vi "IR and Dielectric Strength Test.vi"(0 "VISA resource name in":refnum<visa-resource-name>="COM12", 11 "error in (no error)":errorcluster) -> (2 "Stop Status":bool, 3 "Stop Status":string, 4 "BW 1 Results":T2, 6 "BW 2 Results":T2, 8 "Raw Data ACW BW1":T4, 10 "Raw Data ACW BW2":T3, 13 "BW1 Result Indicators":T1, 14 "BW2 Result Indicators":T1, 15 "error out":errorcluster)   [LabVIEW 2018]
uses:
  Custom Controls/Vitrek State Variable.ctl
  <vilib>/Instr/_visa.llb/VISA Configure Serial Port (Instr).vi
  Door Status Global Variable.vi
panel:
  in  "Insulation Resistance (Mohms)":dbl=100.0 format="%#_13g"
  in  "Dielectric Strength (uA)":dbl=50.0 format="%#_13g"
  out "Test Status":string
  out "Dielectric Strength Voltage - BW2":dbl[](graph)
  out "Dielectric Strength Current - BW2":dbl[](graph)
  out "Dielectric Strength Current - BW1":dbl[](graph)
  out "Dielectric Strength Voltage - BW1":dbl[](graph) caption="Dielectric Strength Voltage Test 1"
  out "Test Results":string
  out "Current Step":string
  in  "Vitrek States":T5=enum."Config ACW Bridgewire 1"
  # "Bridgewire 1"
  # "Bridgewire 2"
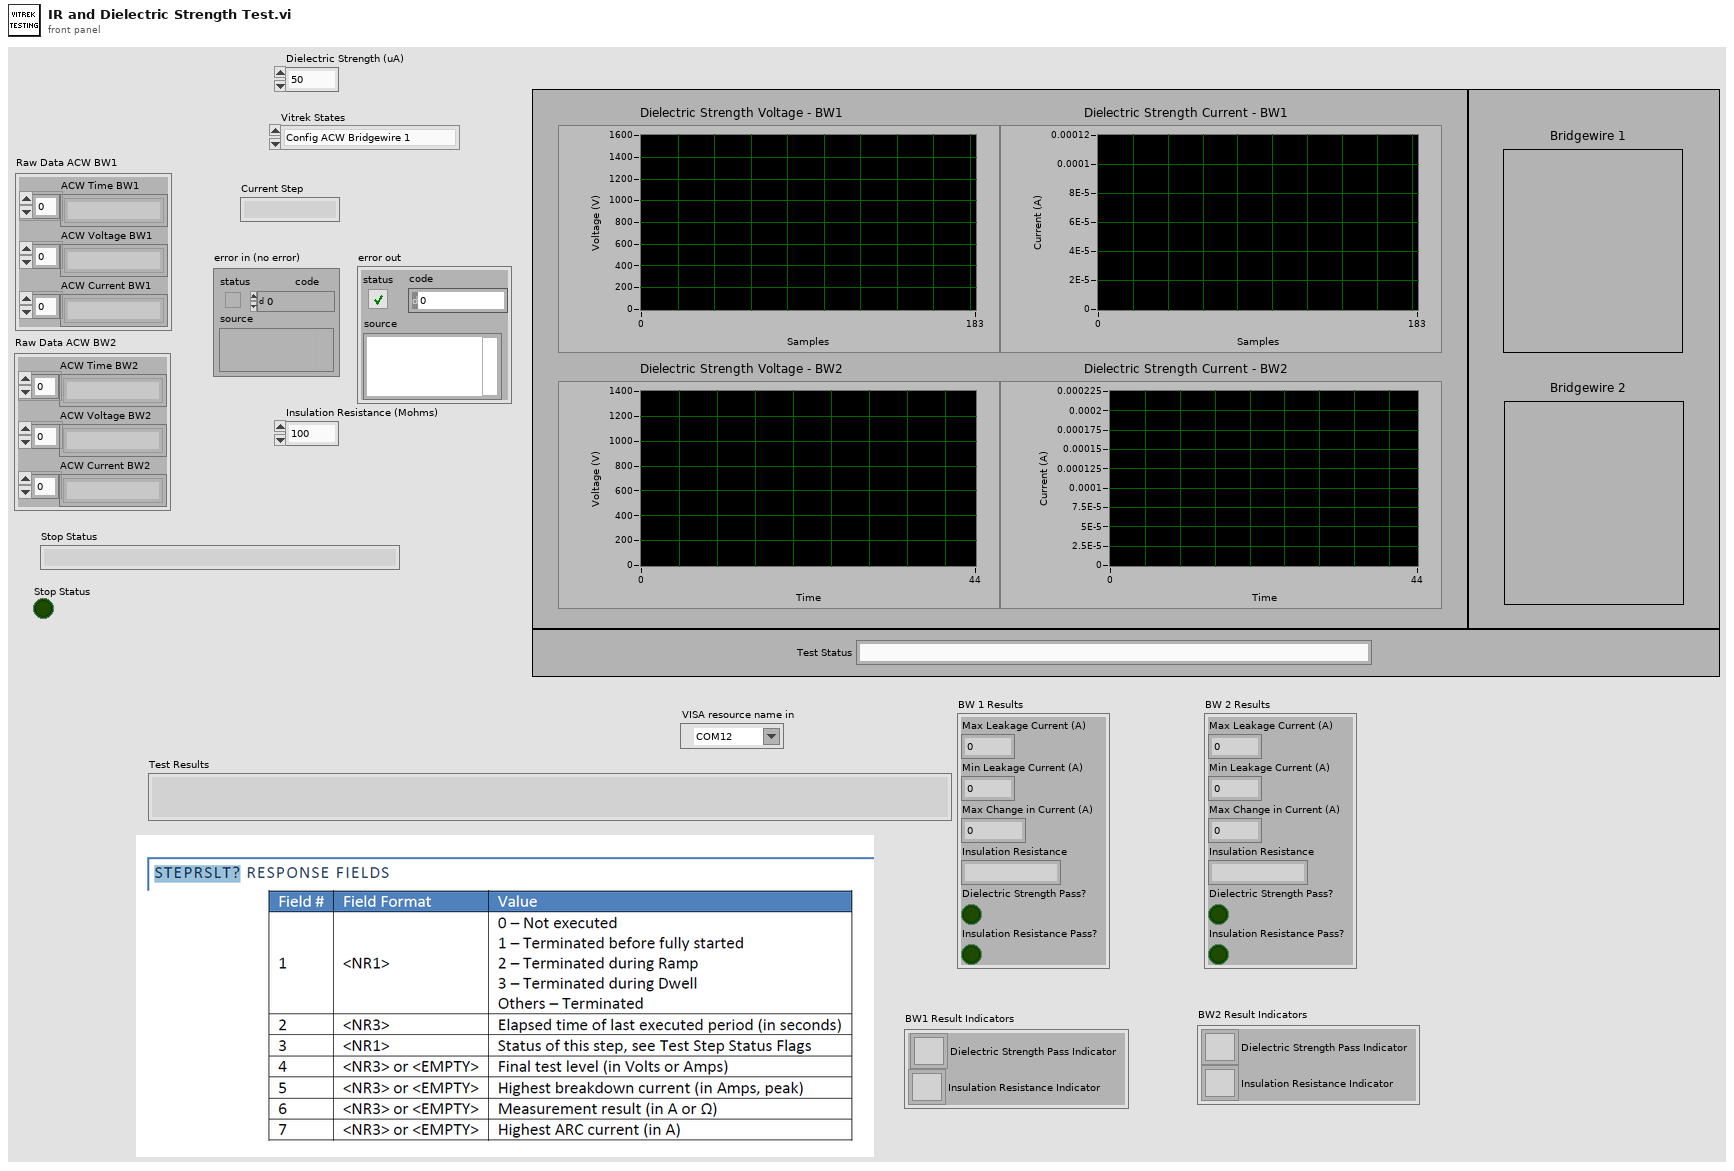
[diagram p1: front panel]
types:
  T1 = cluster{"Dielectric Strength Pass Indicator":u16, "Insulation Resistance Indicator":u16}
  T2 = cluster{"Max Leakage Current (A)":dbl, "Min Leakage Current (A)":dbl, "Max Change in Current (A)":dbl, "Dielectric Strength Pass?":bool, "Insulation Resistance Pass?":bool, "Insulation Resistance":string}
  T3 = cluster{"ACW Time BW2":string[], "ACW Voltage BW2":string[], "ACW Current BW2":string[]}
  T4 = cluster{"ACW Time BW1":string[], "ACW Voltage BW1":string[], "ACW Current BW1":string[]}
  T5 = typedef "Vitrek State Variable.ctl" = enum16{"Clear Tests", "Config ACW Bridgewire 1", "Config ACW Bridgewire 2", "Config IR Bridgewire 1", "Config IR Bridgewire 2", "Run Test", "Stop"}
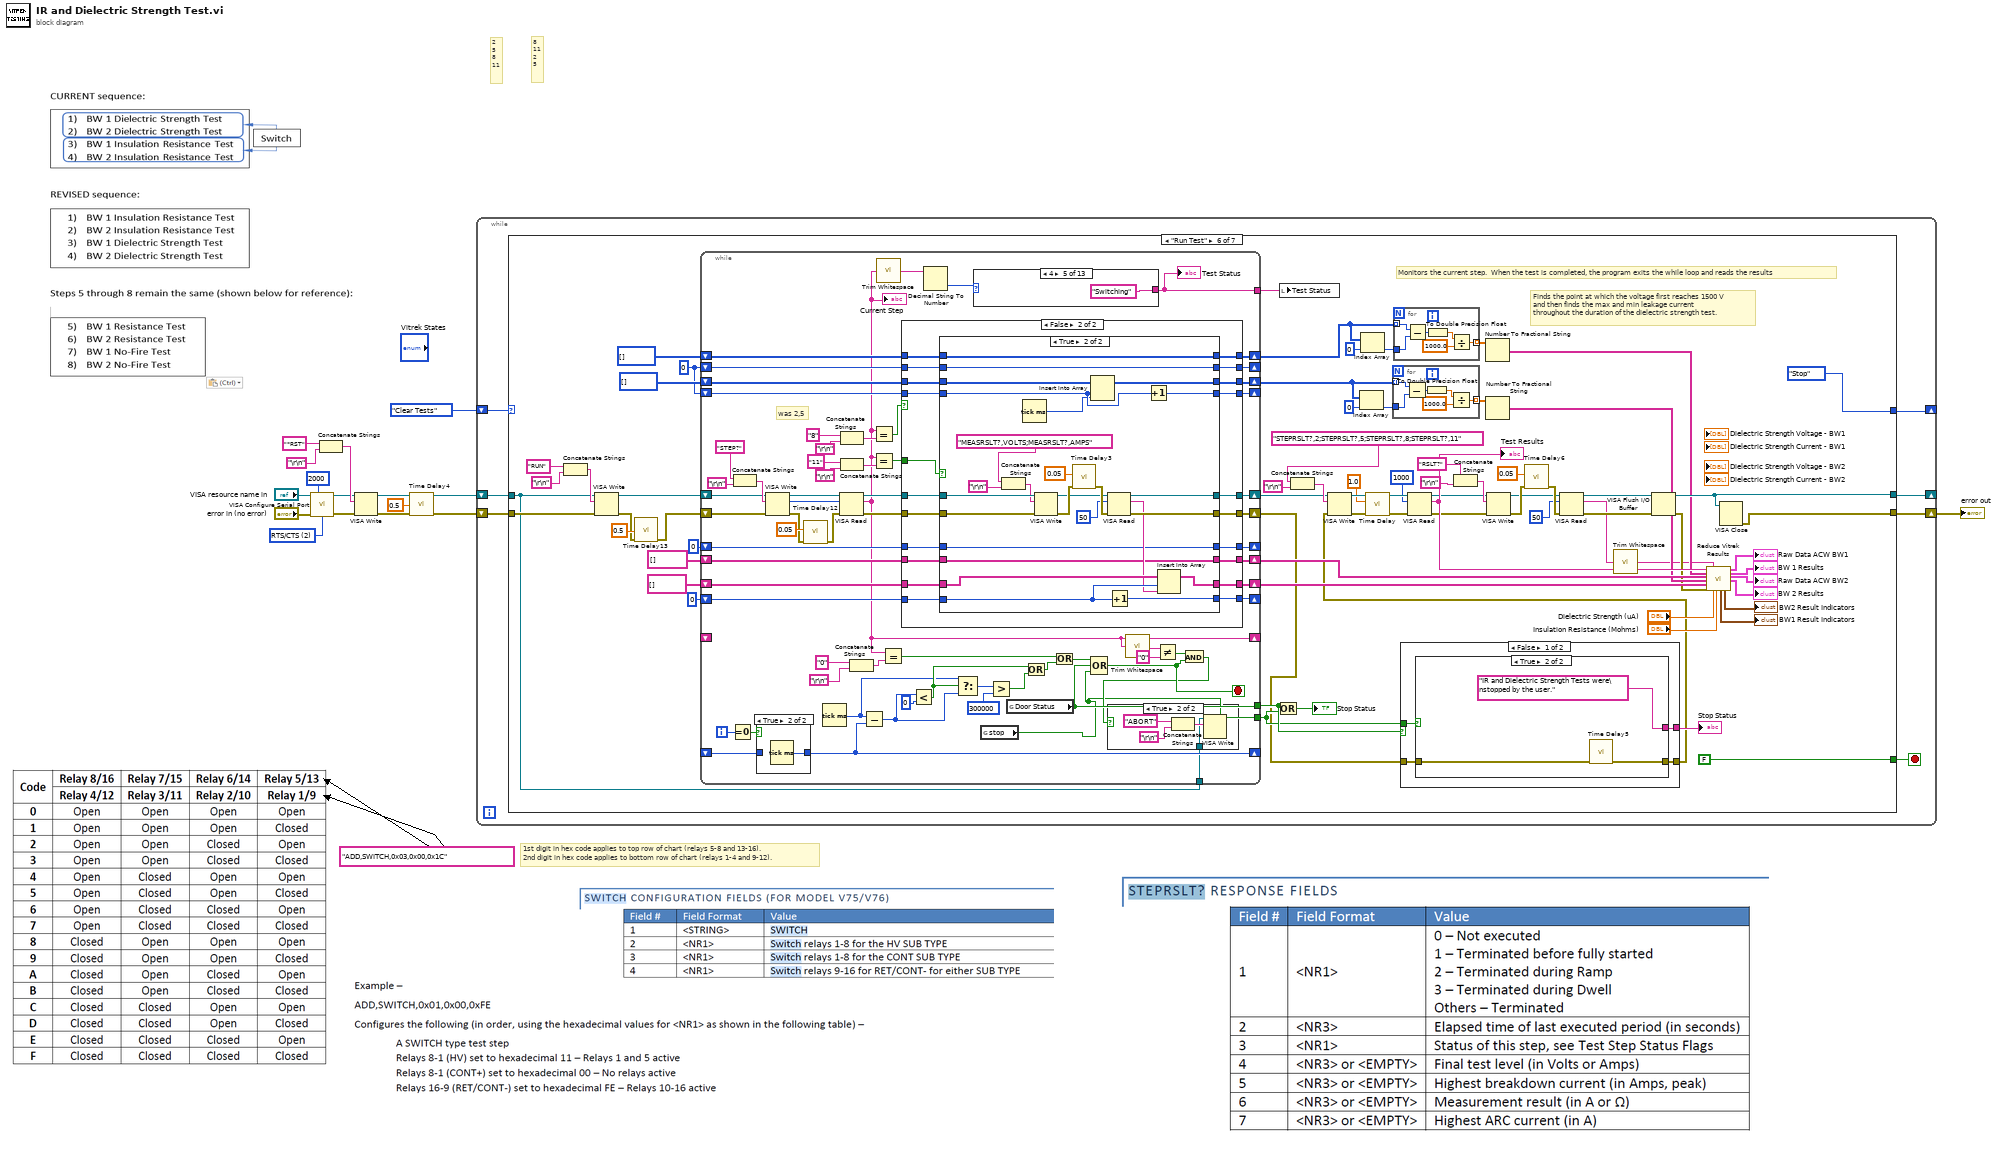
[diagram p0: block diagram]
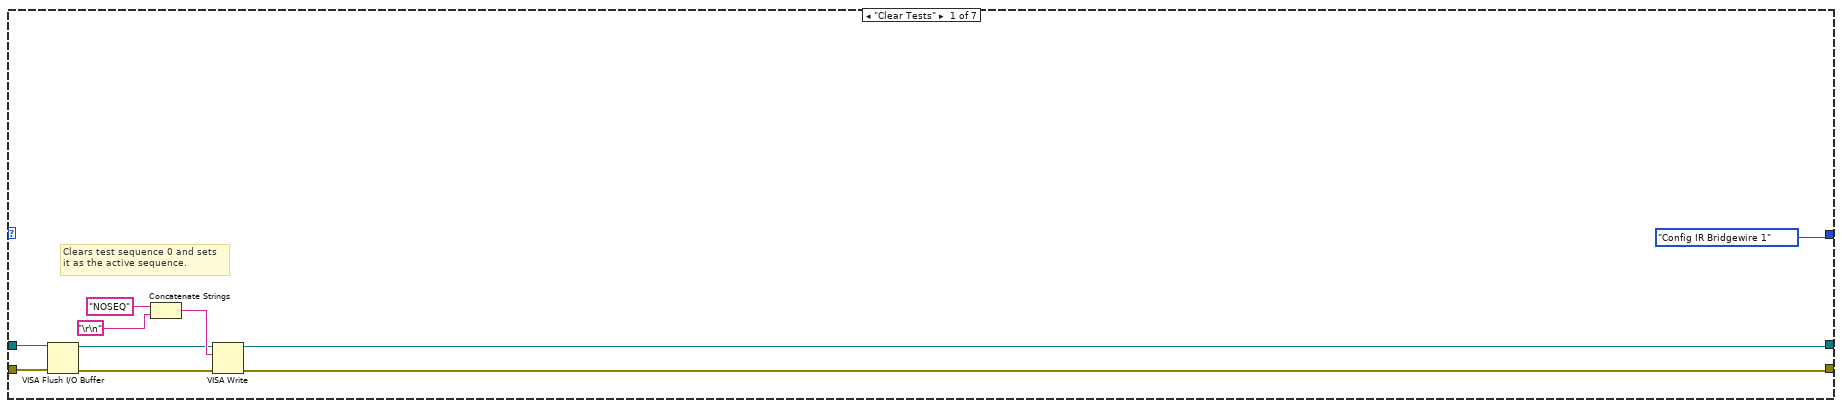
[diagram p2: hidden frame]
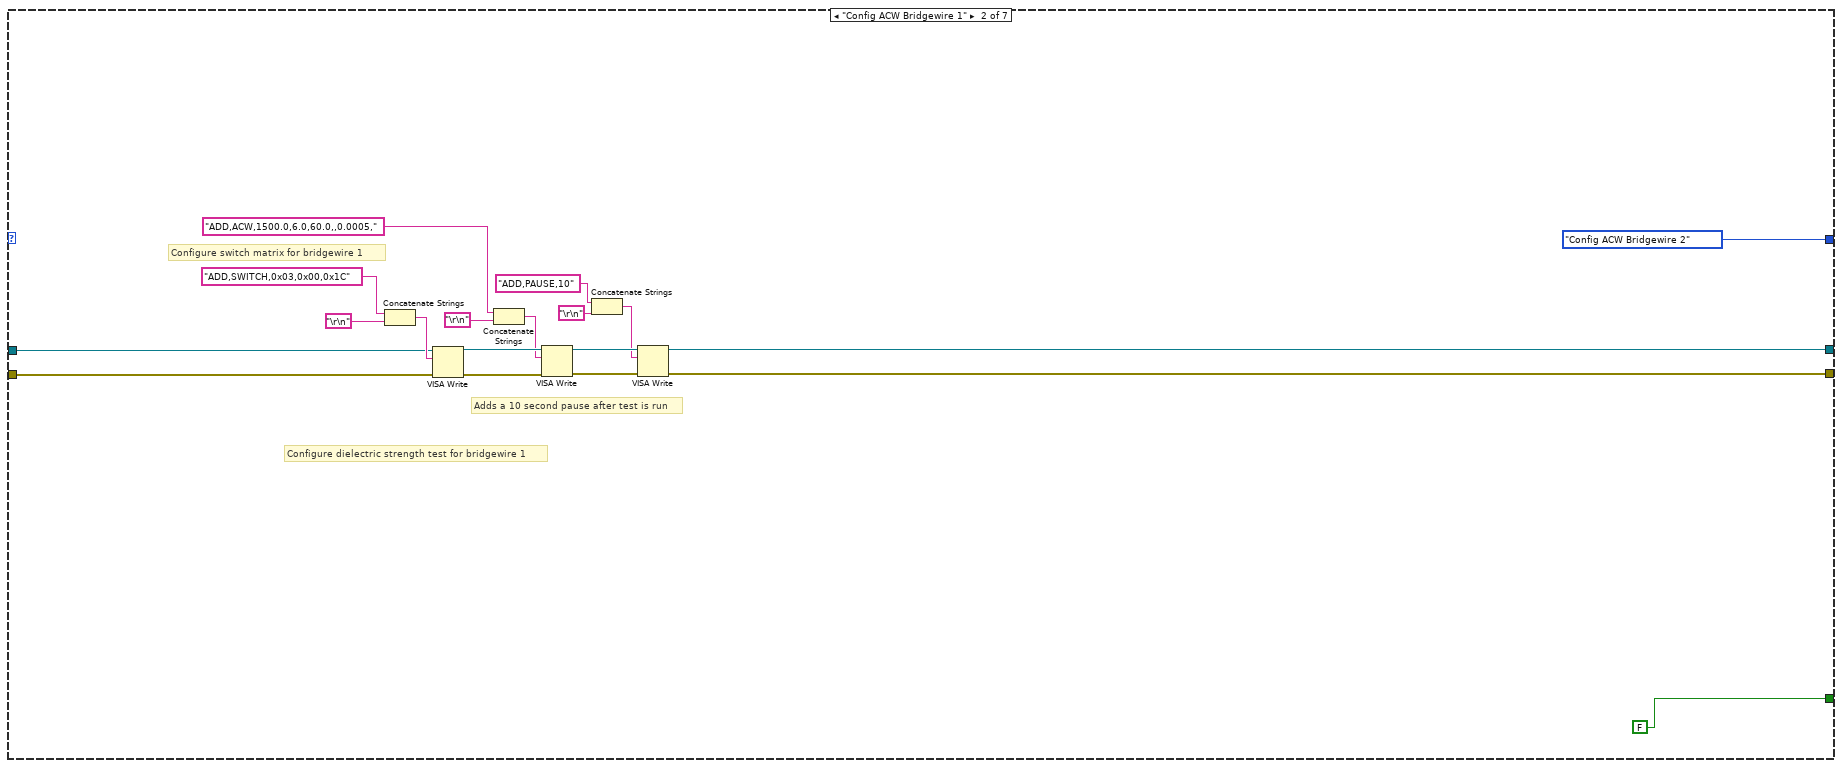
[diagram p3: hidden frame]
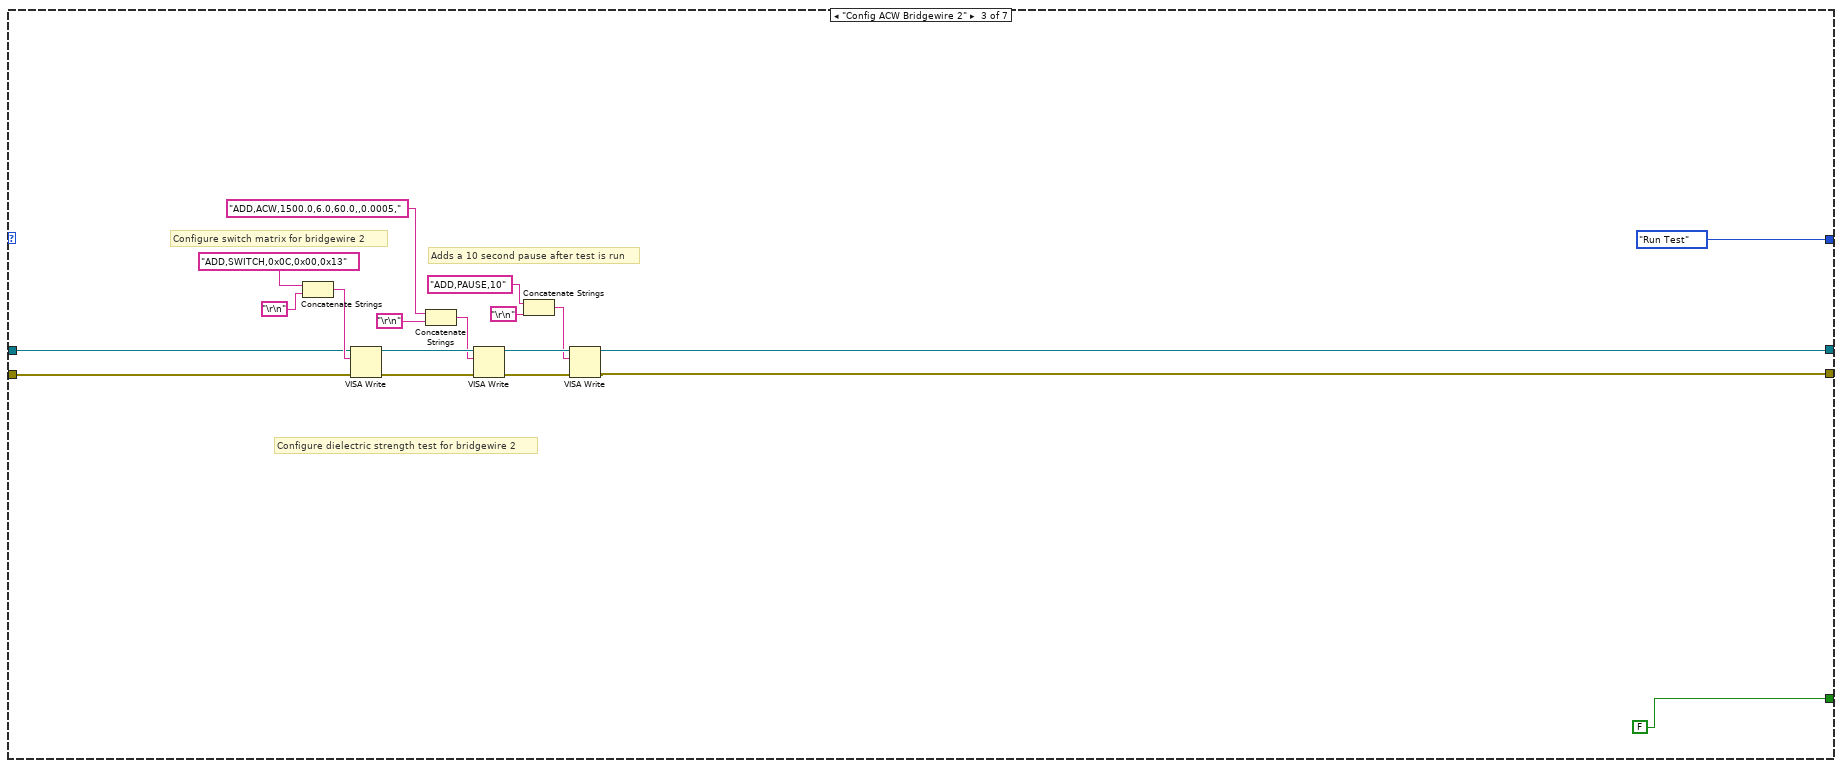
[diagram p4: hidden frame]
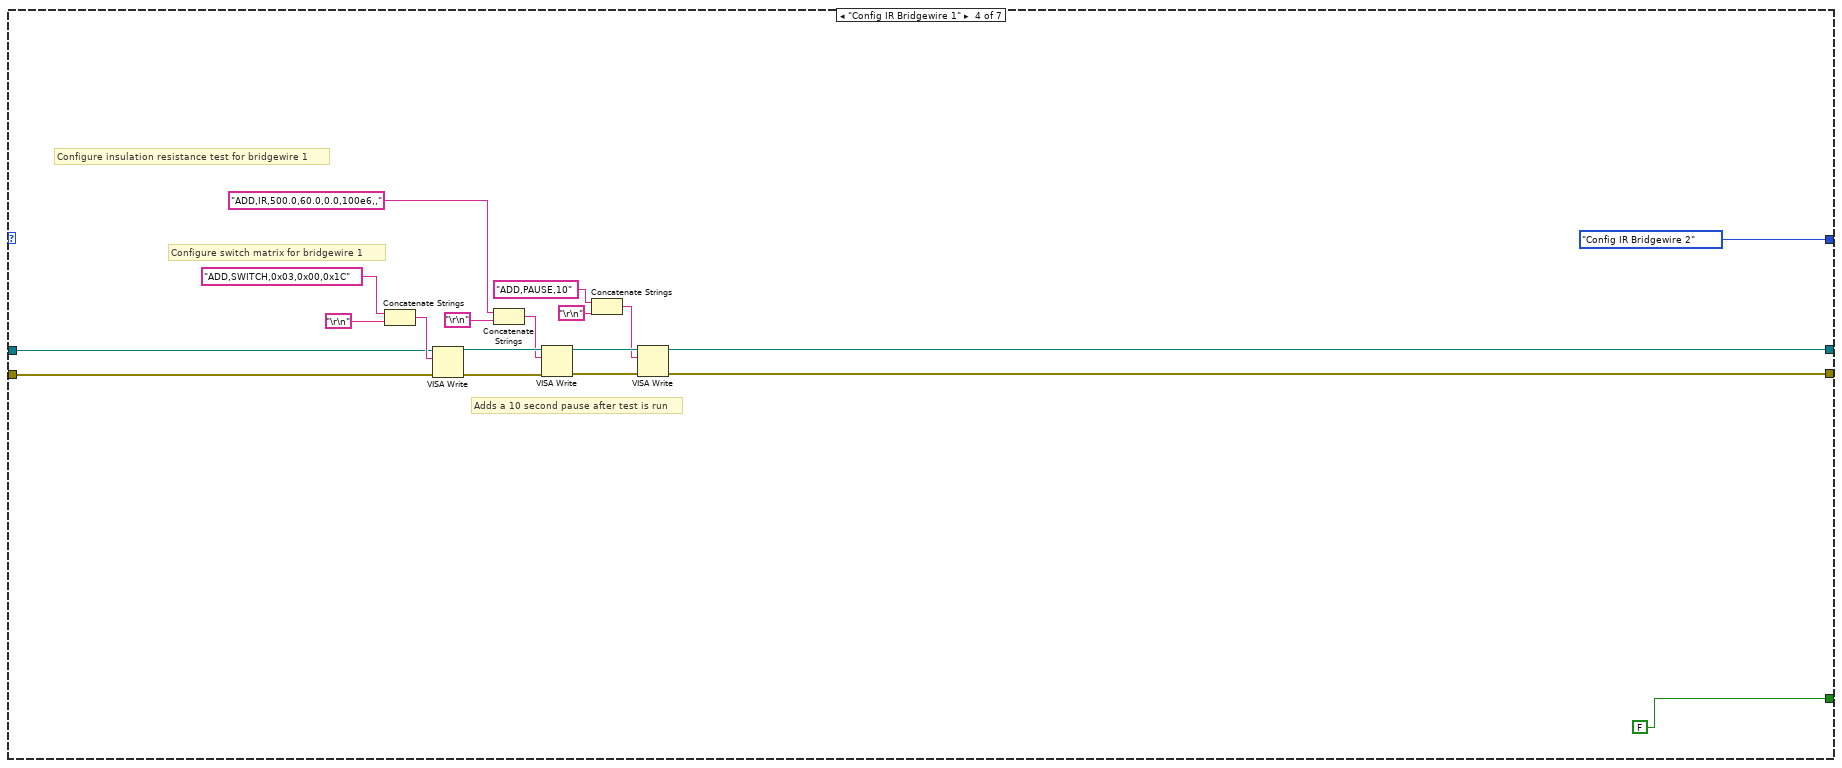
[diagram p5: hidden frame]
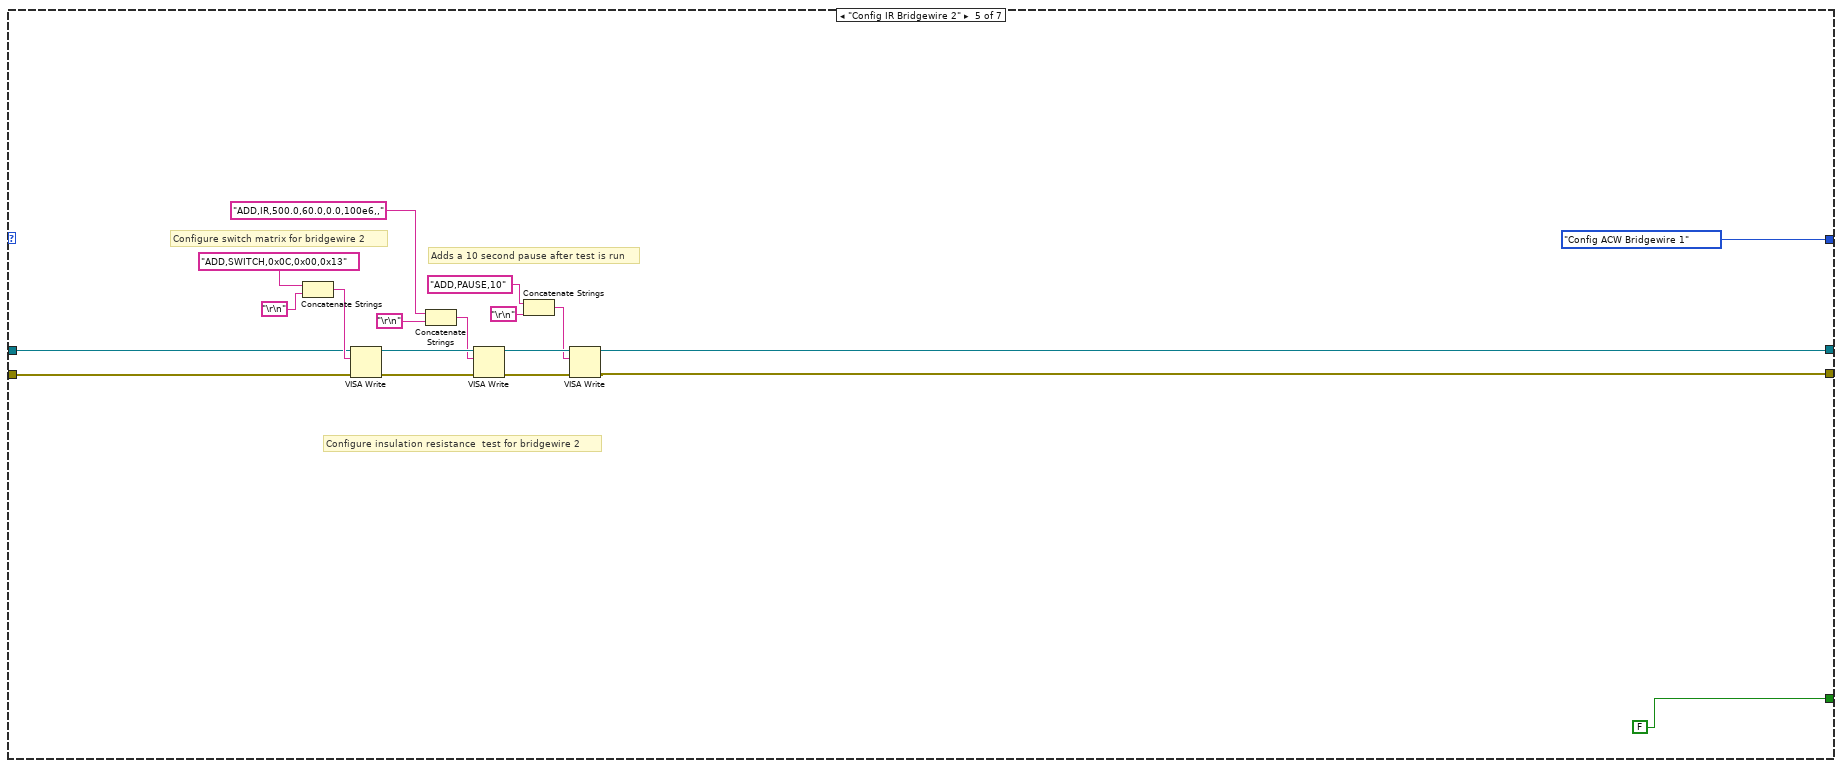
[diagram p6: hidden frame]
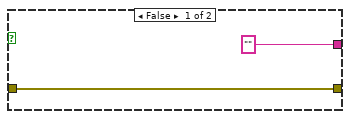
[diagram p7: hidden frame]
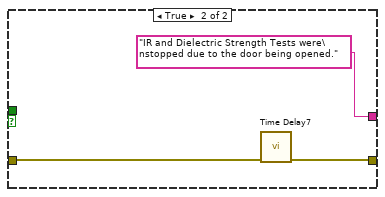
[diagram p8: hidden frame]
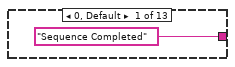
[diagram p10: hidden frame]
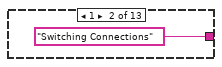
[diagram p11: hidden frame]
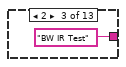
[diagram p12: hidden frame]
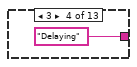
[diagram p13: hidden frame]
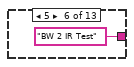
[diagram p14: hidden frame]
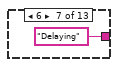
[diagram p15: hidden frame]
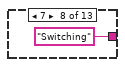
[diagram p16: hidden frame]
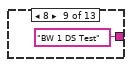
[diagram p17: hidden frame]
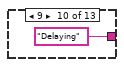
[diagram p18: hidden frame]
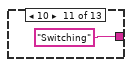
[diagram p19: hidden frame]
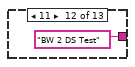
[diagram p20: hidden frame]
diagram:
  (unwired) "ADD,SWITCH,0x03,0x00,0x1C" ("multi-line string")
  w14 = u16 2 items=["None", "XON/XOFF", "RTS/CTS", "XON/XOFF & RTS/CTS", "DTR/DSR", "XON/XOFF & DTR/DSR"] ("flow control (0:none)")
  # "8\n11\n2\n5"
  # "2\n5\n8\n11"
  # "1st digit in hex code applies to top row of chart (relays 5-8 and 13-16).\n2nd digit in hex code applies to bottom row of chart (relays 1-4 and 9-12)."
  n1 = call-poly "VISA Configure Serial Port"("VISA resource name"="VISA resource name in", "timeout (10sec)"=u32 2000, "error in (no error)"="error in (no error)", "flow control (0:none)"=w14) -> ("VISA resource name out"=w9:refnum<visa-resource-name>, "error out"=w10:errorcluster)  [unwired: 10 in]
  n2 = Concatenate Strings("*RST" ("write buffer"), "\r\n") -> (w11:string)
  n3 = VISA Write(VISA resource name=w9, write buffer=w11, error in (no error)=w10) -> (VISA resource name out=w4:refnum<visa-resource-name>, error out=w6:errorcluster)  [unwired: 1 out]
  n4 = call "Time Delay4"("error in (no error)"=w6, "Delay Time (s)"=0.5) -> ("error out"=w3:errorcluster)  [unwired: 9 in]
  n5 = while {
    shift-right: [w18] -> _
    shift-left: w4 -> [w21]
    shift-right: [w17] -> w2
    shift-left: w3 -> [w20]
    shift-right: [w19] -> _
    shift-left: Vitrek_State_Variable."Clear Tests" ("Vitrek States") -> [w22]
    stop <- w16 stop-if-true
    n6 = case shown="\"Run Test\"" w22 {
      tunnel: w21 -> [w27 w34 w53 w75 w91 w109 w375]
      tunnel: w20 -> [w26 w33 w52 w74 w90 w173 w374]
      tunnel: [Vitrek_State_Variable."Config IR Bridgewire 1" ("Vitrek States") Vitrek_State_Variable."Config ACW Bridgewire 2" ("Vitrek States") Vitrek_State_Variable."Run Test" ("Vitrek States") Vitrek_State_Variable."Config IR Bridgewire 2" ("Vitrek States") Vitrek_State_Variable."Config ACW Bridgewire 1" ("Vitrek States") Vitrek_State_Variable."Stop" ("Vitrek States") Vitrek_State_Variable."Stop" ("Vitrek States")] -> w19
      tunnel: [w25 w38 w55 w72 w93 w156 w375] -> w18
      tunnel: [w24 w36 w54 w73 w92 w157 w374] -> w17
      tunnel: [_ FALSE FALSE FALSE FALSE FALSE TRUE] -> w16
      frame "Clear Tests" {
        # "Clears test sequence 0 and sets \nit as the active sequence."
        n7 = VISA Flush I/O Buffer(VISA resource name=w27, error in (no error)=w26) -> (VISA resource name out=w29:refnum<visa-resource-name>, error out=w28:errorcluster)  [unwired: 1 in]
        n8 = Concatenate Strings("NOSEQ" ("write buffer"), "\r\n") -> (w30:string)
        n9 = VISA Write(VISA resource name=w29, write buffer=w30, error in (no error)=w28) -> (VISA resource name out=w25:refnum<visa-resource-name>, error out=w24:errorcluster)  [unwired: 1 out]
      }
      frame "Config ACW Bridgewire 1" {
        # "Adds a 10 second pause after test is run"
        # "Configure dielectric strength test for bridgewire 1"
        # "Configure switch matrix for bridgewire 1"
        n10 = Concatenate Strings("ADD,SWITCH,0x03,0x00,0x1C" ("multi-line string"), "\r\n") -> (w40:string)
        n11 = VISA Write(VISA resource name=w34, write buffer=w40, error in (no error)=w33) -> (VISA resource name out=w42:refnum<visa-resource-name>, error out=w43:errorcluster)  [unwired: 1 out]
        n12 = Concatenate Strings("ADD,ACW,1500.0,6.0,60.0,,0.0005," ("write buffer"), "\r\n") -> (w41:string)
        n13 = VISA Write(VISA resource name=w42, write buffer=w41, error in (no error)=w43) -> (VISA resource name out=w48:refnum<visa-resource-name>, error out=w49:errorcluster)  [unwired: 1 out]
        n14 = Concatenate Strings("ADD,PAUSE,10" ("write buffer"), "\r\n") -> (w47:string)
        n15 = VISA Write(VISA resource name=w48, write buffer=w47, error in (no error)=w49) -> (VISA resource name out=w38:refnum<visa-resource-name>, error out=w36:errorcluster)  [unwired: 1 out]
      }
      frame "Config ACW Bridgewire 2" {
        # "Adds a 10 second pause after test is run"
        # "Configure dielectric strength test for bridgewire 2"
        # "Configure switch matrix for bridgewire 2"
        n16 = Concatenate Strings("ADD,SWITCH,0x0C,0x00,0x13" ("multi-line string"), "\r\n") -> (w59:string)
        n17 = VISA Write(VISA resource name=w53, write buffer=w59, error in (no error)=w52) -> (VISA resource name out=w61:refnum<visa-resource-name>, error out=w62:errorcluster)  [unwired: 1 out]
        n18 = Concatenate Strings("ADD,ACW,1500.0,6.0,60.0,,0.0005," ("write buffer"), "\r\n") -> (w60:string)
        n19 = VISA Write(VISA resource name=w61, write buffer=w60, error in (no error)=w62) -> (VISA resource name out=w67:refnum<visa-resource-name>, error out=w68:errorcluster)  [unwired: 1 out]
        n20 = Concatenate Strings("ADD,PAUSE,10" ("write buffer"), "\r\n") -> (w66:string)
        n21 = VISA Write(VISA resource name=w67, write buffer=w66, error in (no error)=w68) -> (VISA resource name out=w55:refnum<visa-resource-name>, error out=w54:errorcluster)  [unwired: 1 out]
      }
      frame "Config IR Bridgewire 1" {
        # "Adds a 10 second pause after test is run"
        # "Configure insulation resistance test for bridgewire 1"
        # "Configure switch matrix for bridgewire 1"
        n22 = Concatenate Strings("ADD,SWITCH,0x03,0x00,0x1C" ("multi-line string"), "\r\n") -> (w79:string)
        n23 = VISA Write(VISA resource name=w75, write buffer=w79, error in (no error)=w74) -> (VISA resource name out=w81:refnum<visa-resource-name>, error out=w82:errorcluster)  [unwired: 1 out]
        n24 = Concatenate Strings("ADD,IR,500.0,60.0,0.0,100e6,," ("write buffer"), "\r\n") -> (w80:string)
        n25 = VISA Write(VISA resource name=w81, write buffer=w80, error in (no error)=w82) -> (VISA resource name out=w86:refnum<visa-resource-name>, error out=w87:errorcluster)  [unwired: 1 out]
        n26 = Concatenate Strings("ADD,PAUSE,10" ("write buffer"), "\r\n") -> (w85:string)
        n27 = VISA Write(VISA resource name=w86, write buffer=w85, error in (no error)=w87) -> (VISA resource name out=w72:refnum<visa-resource-name>, error out=w73:errorcluster)  [unwired: 1 out]
      }
      frame "Config IR Bridgewire 2" {
        # "Adds a 10 second pause after test is run"
        # "Configure insulation resistance  test for bridgewire 2"
        # "Configure switch matrix for bridgewire 2"
        n28 = Concatenate Strings("ADD,SWITCH,0x0C,0x00,0x13" ("multi-line string"), "\r\n") -> (w97:string)
        n29 = VISA Write(VISA resource name=w91, write buffer=w97, error in (no error)=w90) -> (VISA resource name out=w99:refnum<visa-resource-name>, error out=w100:errorcluster)  [unwired: 1 out]
        n30 = Concatenate Strings("ADD,IR,500.0,60.0,0.0,100e6,," ("write buffer"), "\r\n") -> (w98:string)
        n31 = VISA Write(VISA resource name=w99, write buffer=w98, error in (no error)=w100) -> (VISA resource name out=w105:refnum<visa-resource-name>, error out=w106:errorcluster)  [unwired: 1 out]
        n32 = Concatenate Strings("ADD,PAUSE,10" ("write buffer"), "\r\n") -> (w104:string)
        n33 = VISA Write(VISA resource name=w105, write buffer=w104, error in (no error)=w106) -> (VISA resource name out=w93:refnum<visa-resource-name>, error out=w92:errorcluster)  [unwired: 1 out]
      }
      frame "Run Test" {
        w126 = 0 ("index")
        # "Finds the point at which the voltage first reaches 1500 V\nand then finds the max and min leakage current \nthroughout the duration of the dielectric strength test."
        # "Monitors the current step.  When the test is completed, the program exits the while loop and reads the results"
        n34 = Concatenate Strings("RUN" ("write buffer"), "\r\n") -> (w176:string)
        n35 = VISA Write(VISA resource name=w109, write buffer=w176, error in (no error)=w173) -> (VISA resource name out=w175:refnum<visa-resource-name>, error out=w179:errorcluster)  [unwired: 1 out]
        n36 = call "Time Delay13"("error in (no error)"=w179, "Delay Time (s)"=0.5) -> ("error out"=w174:errorcluster)  [unwired: 9 in]
        n37 = while {
          shift-right: [w237] -> w111
          shift-left: w174 -> [w247]
          shift-right: [w232] -> w141
          shift-left: w175 -> [w246]
          shift-right: [w257] -> _
          shift-left: _ -> [w255]
          shift-right: [w233] -> w138
          shift-left: string[] [] -> [w236]
          shift-right: [w234] -> w136
          shift-left: string[] [] -> [w235]
          shift-right: [w230] -> _
          shift-left: 0 ("index") -> [w231]
          shift-right: [w228] -> _
          shift-left: 0 ("index") -> [w229]
          tunnel: [w227] -> w158
          shift-right: [w224] -> w151
          shift-left: u32[] [] -> [w223]
          shift-right: [w222] -> w148
          shift-left: u32[] [] -> [w225]
          shift-right: [w218] -> _
          shift-left: w126 -> [w221]
          shift-right: [w220] -> _
          shift-left: w126 -> [w219]
          tunnel: [w216] -> w145
          tunnel: [w209] -> w144
          shift-right: [w208] -> _
          shift-left: _ -> [_]
          tunnel: w109 -> [w210]
          i -> [w259]
          stop <- w212 stop-if-true
          # "was 2,5"
          n38 = Equal To 0?(x=w259) -> (x = 0?=w258:bool)
          n39 = Concatenate Strings("STEP?" ("write buffer"), "\r\n") -> (w265:string)
          n40 = case shown="True" w258 {
            tunnel: [w372 w373] -> w257
            tunnel: w255 -> [w372 _]
            frame False {
            }
            frame True {
              n41 = Tick Count (ms)() -> (millisecond timer value=w373:u32)
            }
          }
          n42 = VISA Write(VISA resource name=w246, write buffer=w265, error in (no error)=w247) -> (VISA resource name out=w264:refnum<visa-resource-name>, return count=w268:u32, error out=w269:errorcluster)
          n43 = call "Time Delay12"("error in (no error)"=w269, "Delay Time (s)"=0.05) -> ("error out"=w270:errorcluster)  [unwired: 9 in]
          n44 = Tick Count (ms)() -> (millisecond timer value=w250:u32)
          n45 = VISA Read(VISA resource name=w264, byte count=w268, error in (no error)=w270) -> (VISA resource name out=w239:refnum<visa-resource-name>, read buffer=w208:string, error out=w238:errorcluster)  [unwired: 1 out]
          "Current Step" <- w208
          n46 = Concatenate Strings("8", "\r\n") -> (w240:string)
          n47 = Concatenate Strings("11", "\r\n") -> (w245:string)
          n48 = Concatenate Strings("0", "\r\n") -> (w261:string)
          n49 = Subtract(x=w250, y=w257) -> (x-y=w249:u32)
          n50 = Equal?(x=w208, y=w240) -> (x = y?=w206:bool)
          n51 = Equal?(x=w208, y=w245) -> (x = y?=w205:bool)
          n52 = call <vilib>:"Trim Whitespace.vi"("string"=w208) -> ("trimmed string"=w207:string)  [unwired: 1 in]
          n53 = Equal?(x=w208, y=w261) -> (x = y?=w260:bool)
          n54 = case shown="False" w206 {
            tunnel: w239 -> [w306 w334]
            tunnel: w238 -> [w307 w335]
            tunnel: [w304 w333] -> w237
            tunnel: w236 -> [w303 w316]
            tunnel: w235 -> [w300 w332]
            tunnel: [w300 w331] -> w234
            tunnel: [w301 w315] -> w233
            tunnel: [w299 w330] -> w232
            tunnel: w231 -> [w298 w318]
            tunnel: [w297 w317] -> w230
            tunnel: w229 -> [w296 w329]
            tunnel: [w296 w328] -> w228
            tunnel: w225 -> [w290 w327]
            tunnel: [w293 w322] -> w224
            tunnel: w223 -> [w294 w323]
            tunnel: [w290 w326] -> w222
            tunnel: w221 -> [w289 w325]
            tunnel: [w291 w320] -> w220
            tunnel: w219 -> [w292 w321]
            tunnel: [w289 w324] -> w218
            tunnel: w205 -> [_ w319]
            frame True {
              n55 = Concatenate Strings("MEASRSLT?,VOLTS;MEASRSLT?,AMPS" ("write buffer"), "\r\n") -> (w312:string)
              n56 = VISA Write(VISA resource name=w306, write buffer=w312, error in (no error)=w307) -> (VISA resource name out=w311:refnum<visa-resource-name>, error out=w313:errorcluster)  [unwired: 1 out]
              n57 = Tick Count (ms)() -> (millisecond timer value=w295:u32)
              n58 = call "Time Delay2"("error in (no error)"=w313, "Delay Time (s)"=0.05) -> ("error out"=w314:errorcluster)  [unwired: 9 in]
              n59 = Insert Into Array(array=w294, index=w292, new element=w295) -> (w293:u32[])
              n60 = VISA Read(VISA resource name=w311, byte count=u32 50, error in (no error)=w314) -> (VISA resource name out=w299:refnum<visa-resource-name>, read buffer=w302:string, error out=w304:errorcluster)  [unwired: 1 out]
              n61 = Increment(x=w292) -> (x+1=w291:i32)
              n62 = Insert Into Array(array=w303, index=w298, new element=w302) -> (w301:string[])
              n63 = Increment(x=w298) -> (x+1=w297:i32)
            }
            frame False {
              n64 = case shown="True" w319 {
                tunnel: w335 -> [w340 w371]
                tunnel: w334 -> [w341 w370]
                tunnel: [w340 w369] -> w333
                tunnel: w332 -> [w337 w368]
                tunnel: [w337 w367] -> w331
                tunnel: [w341 w366] -> w330
                tunnel: w329 -> [w336 w365]
                tunnel: [w336 w364] -> w328
                tunnel: w327 -> [w343 w363]
                tunnel: [w343 w362] -> w326
                tunnel: w325 -> [w342 w361]
                tunnel: [w342 w360] -> w324
                tunnel: w321 -> [w344 w348]
                tunnel: w323 -> [w345 w349]
                tunnel: [w345 w349] -> w322
                tunnel: [w344 w348] -> w320
                tunnel: w318 -> [w339 w347]
                tunnel: [w339 w347] -> w317
                tunnel: w316 -> [w338 w346]
                tunnel: [w338 w346] -> w315
                frame False {
                }
                frame True {
                  n65 = Concatenate Strings("MEASRSLT?,VOLTS;MEASRSLT?,AMPS" ("write buffer"), "\r\n") -> (w357:string)
                  n66 = Tick Count (ms)() -> (millisecond timer value=w350:u32)
                  n67 = VISA Write(VISA resource name=w370, write buffer=w357, error in (no error)=w371) -> (VISA resource name out=w356:refnum<visa-resource-name>, error out=w358:errorcluster)  [unwired: 1 out]
                  n68 = call "Time Delay3"("error in (no error)"=w358, "Delay Time (s)"=0.05) -> ("error out"=w359:errorcluster)  [unwired: 9 in]
                  n69 = Insert Into Array(array=w363, index=w361, new element=w350) -> (w362:u32[])
                  n70 = VISA Read(VISA resource name=w356, byte count=u32 50, error in (no error)=w359) -> (VISA resource name out=w366:refnum<visa-resource-name>, read buffer=w351:string, error out=w369:errorcluster)  [unwired: 1 out]
                  n71 = Increment(x=w365) -> (x+1=w364:i32)
                  n72 = Increment(x=w361) -> (x+1=w360:i32)
                  n73 = Insert Into Array(array=w368, index=w365, new element=w351) -> (w367:string[])
                }
              }
            }
          }
          n74 = Less?(x=w249, y=u32 0) -> (x < y?=w251:bool)
          n75 = Decimal String To Number(string=w207) -> (number=w226:i32)  [unwired: 2 in, 1 out]
          n76 = Select(t=w250, s=w251, f=w249) -> (s? t:f=w248:u32)
          n77 = case shown="4" w226 {
            tunnel: ["Sequence Completed" ("Test Status") "Switching Connections" ("Test Status") "BW IR Test" ("Test Status") "Delaying" ("Test Status") "Switching" ("Test Status") "BW 2 IR Test" ("Test Status") "Delaying" ("Test Status") "Switching" ("Test Status") "BW 1 DS Test" ("Test Status") "Delaying" ("Test Status") "Switching" ("Test Status") "BW 2 DS Test" ("Test Status") "Delaying" ("Test Status")] -> w227
            frame 0, Default {
            }
            frame 1 {
            }
            frame 2 {
            }
            frame 3 {
            }
            frame 4 {
            }
            frame 5 {
            }
            frame 6 {
            }
            frame 7 {
            }
            frame 8 {
            }
            frame 9 {
            }
            frame 10 {
            }
            frame 11 {
            }
            frame 12 {
            }
          }
          "Test Status" <- w227
          n78 = global read "Door Status Global Variable.vi" "stop"() -> (w209:bool)
          n79 = Greater?(x=w248, y=u32 300000) -> (0:w253:bool)
          n80 = global read "Door Status Global Variable.vi" "Door Status"() -> (w216:bool)
          n81 = Or(x=w251, y=w253) -> (x .or. y?=w252:bool)
          n82 = Or(x=w260, y=w252) -> (x .or. y?=w217:bool)
          n83 = Compound Arithmetic op=OR(w217, w216, w209) -> (w212:bool)
          n84 = call <vilib>:"Trim Whitespace.vi"("string"=w208) -> ("trimmed string"=w215:string)  [unwired: 1 in]
          n85 = Not Equal?(x=w215, y="0") -> (x != y?=w213:bool)
          n86 = And(x=w213, y=w212) -> (x .and. y?=w211:bool)
          n87 = case shown="True" w211 {
            tunnel: w210 -> [_ w272]
            frame False {
            }
            frame True {
              n88 = Concatenate Strings("ABORT" ("write buffer"), "\r\n") -> (w275:string)
              n89 = VISA Write(VISA resource name=w272, write buffer=w275) -> ()  [unwired: 1 in, 3 out]
            }
          }
        }
        n90 = Or(x=w145, y=w144) -> (x .or. y?=→"Stop Status":bool)
        n91 = local write "Test Status"(w158) -> ()
        n92 = Concatenate Strings("STEPRSLT?,2;STEPRSLT?,5;STEPRSLT?,8;STEPRSLT?,11" ("write buffer"), "\r\n") -> (w169:string)
        n93 = Index Array(array=w148, index=0) -> (element=w150:u32)
        n94 = Index Array(array=w151, index=0) -> (element=w154:u32)
        n95 = for {
          tunnel: w150 -> [w194]
          tunnel: [w195] -> w146 mode=indexing
          tunnel: w148 -> [w193] mode=indexing
          n96 = Subtract(x=w193, y=w194) -> (x-y=w198:u32)
          n97 = To Double Precision Float(number=w198) -> (double precision float=w197:dbl)
          n98 = Divide(x=w197, y=1000.0) -> (x/y=w195:dbl)
        }
        n99 = for {
          tunnel: w154 -> [w200]
          tunnel: [w201] -> w147 mode=indexing
          tunnel: w151 -> [w199] mode=indexing
          n100 = Subtract(x=w199, y=w200) -> (x-y=w204:u32)
          n101 = To Double Precision Float(number=w204) -> (double precision float=w203:dbl)
          n102 = Divide(x=w203, y=1000.0) -> (x/y=w201:dbl)
        }
        n103 = case shown="False" w145 {
          tunnel: [w184 "IR and Dielectric Strength Tests were\nstopped due to the door being opened." ("Test Status")] -> w142
          tunnel: w144 -> [w183 _]
          tunnel: w111 -> [w182 w190]
          tunnel: [w181 w191] -> w110
          frame False {
            n104 = case shown="True" w183 {
              tunnel: ["" ("Test Status") "IR and Dielectric Strength Tests were\nstopped by the user." ("Test Status")] -> w184
              tunnel: w182 -> [w185 w187]
              tunnel: [w185 w188] -> w181
              frame False {
              }
              frame True {
                n105 = call "Time Delay5"("error in (no error)"=w187) -> ("error out"=w188:errorcluster)  [unwired: 10 in]
              }
            }
          }
          frame True {
            n106 = call "Time Delay7"("error in (no error)"=w190) -> ("error out"=w191:errorcluster)  [unwired: 10 in]
          }
        }
        "Stop Status" <- w142
        n107 = VISA Write(VISA resource name=w141, write buffer=w169, error in (no error)=w110) -> (VISA resource name out=w170:refnum<visa-resource-name>, error out=w166:errorcluster)  [unwired: 1 out]
        n108 = call "Time Delay"("error in (no error)"=w166, "Delay Time (s)"=1.0) -> ("error out"=w165:errorcluster)  [unwired: 9 in]
        n109 = VISA Read(VISA resource name=w170, byte count=u32 1000, error in (no error)=w165) -> (VISA resource name out=w116:refnum<visa-resource-name>, read buffer=w140:string, error out=w117:errorcluster)  [unwired: 1 out]
        "Test Results" <- w140
        n110 = Concatenate Strings("RSLT?" ("write buffer"), "\r\n") -> (w123:string)
        n111 = Number To Fractional String(number=w147) -> (F-format string=w139:string[])  [unwired: 3 in]
        n112 = Number To Fractional String(number=w146) -> (F-format string=w137:string[])  [unwired: 3 in]
        n113 = VISA Write(VISA resource name=w116, write buffer=w123, error in (no error)=w117) -> (VISA resource name out=w122:refnum<visa-resource-name>, error out=w124:errorcluster)  [unwired: 1 out]
        n114 = call "Time Delay6"("error in (no error)"=w124, "Delay Time (s)"=0.05) -> ("error out"=w125:errorcluster)  [unwired: 9 in]
        n115 = VISA Read(VISA resource name=w122, byte count=u32 50, error in (no error)=w125) -> (VISA resource name out=w115:refnum<visa-resource-name>, read buffer=w113:string, error out=w114:errorcluster)  [unwired: 1 out]
        n116 = call <vilib>:"Trim Whitespace.vi"("string"=w113) -> ("trimmed string"=w112:string)  [unwired: 1 in]
        n117 = VISA Flush I/O Buffer(VISA resource name=w115, error in (no error)=w114) -> (VISA resource name out=w156:refnum<visa-resource-name>, error out=w131:errorcluster)  [unwired: 1 in]
        n118 = call "Reduce Vitrek Results.vi"("Results String"=w140, "BW1 ACW Time"=w139, "BW1 ACW Raw"=w138, "BW2 ACW Time"=w137, "BW2 ACW Raw"=w136, "error in (no error)"=w131, "Result Error Status"=w112, "Dielectric Strength Spec (uA)"="Dielectric Strength (uA)", "Insulation Resistance Spec (Mohms)"="Insulation Resistance (Mohms)") -> ("BW1 Results Indicator"=→"BW1 Result Indicators":T1, "BW2 Results Indicator"=→"BW2 Result Indicators":T1, "Raw Data ACW BW1"=→"Raw Data ACW BW1":T4, "BW 1 Results"=→"BW 1 Results":T2, "Raw Data ACW BW2"=→"Raw Data ACW BW2":T3, "BW 2 Results"=→"BW 2 Results":T2)  [unwired: 4 in, 1 out]
        n119 = VISA Close(VISA resource name=w156) -> (error out=w157:errorcluster)  [unwired: 1 in]
      }
      frame "Stop" {
      }
    }
  }
  "error out" <- w2
